vi "Validate Attributes JSON.vi"(6 "$Path":string="$.Attributes", 8 "error in":errorcluster, 10 "Cluster in":variant, 11 "<JSON>":string) -> (0 "error out":errorcluster, 2 "<JSON>":string)   [LabVIEW 2023]
uses:
  b690fbb4-b114-4137-a40c-faf688a51290.vi
  <vilib>/JDP Science/JSONtext/Next JSON Value.vi
  <vilib>/JDP Science/JSONtext/String Subset.vi
  <vilib>/JDP Science/JSONtext/Parsing/Advance past next JSON Value (inlined COPY).vi
  <vilib>/JDP Science/JSONtext/Parsing/Advance past whitespace.vi
  <vilib>/JDP Science/JSONtext/Parsing/Advance past String.vi
  <vilib>/JDP Science/JSONtext/Parsing/Advance past Number.vi
  <vilib>/JDP Science/JSONtext/Parsing/Advance past Line Ending.vi
  <vilib>/JDP Science/JSONtext/Variant to JSON Text.vi
  <vilib>/JDP Science/JSONtext/Parsing/Parse Full Path or Item Name.vi
  <vilib>/JDP Science/JSONtext/Parsing/Advance past Array.vi
  <vilib>/JDP Science/JSONtext/Parsing/Advance past Object.vi
  <vilib>/JDP Science/JSONtext/support/Error Cluster From Code.vi
  <vilib>/JDP Science/JSONtext/Offset/Find Item Locations by Path.vi
  <vilib>/JDP Science/JSONtext/LVClass Serializer/JSONtext LVClass Serializer.lvclass
  <vilib>/JDP Science/JSONtext/JSONtext.lvlib
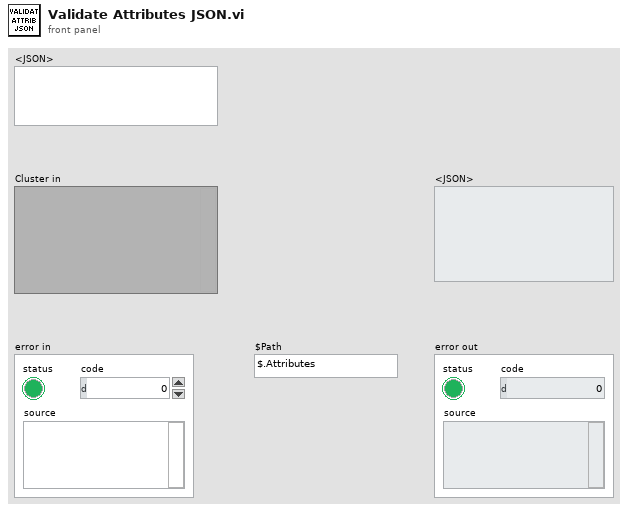
[diagram p1: front panel]
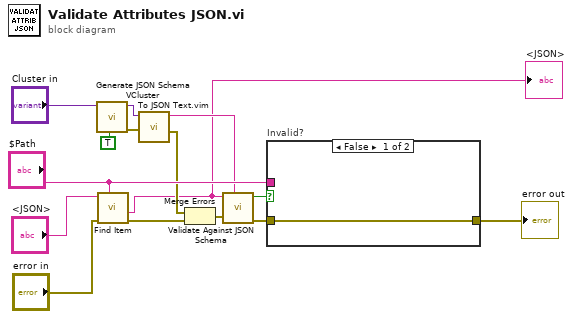
[diagram p0: block diagram]
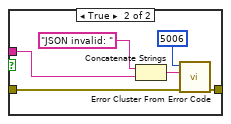
[diagram p2: hidden frame]
diagram:
  n1 = call "Generate JSON Schema VCluster.vi"("strict?"=TRUE, "type"="Cluster in") -> ("error out"=w6:errorcluster, "json schema cluster"=w5:variant)  [unwired: 8 in]
  n2 = call <vilib>:"Find Item.vi"("$Path or Item Name"="$Path", "error in (no error)"="error in", "JSON"="<JSON>") -> ("error out"=w11:errorcluster, "<JSON>"=w1:string)  [unwired: 5 in, 2 out]
  "<JSON>" <- w1
  n3 = call "To JSON Text.vim"("error in (no error)"=w6, "Anything"=w5) -> ("error out"=w8:errorcluster, "<JSON>"=w9:string)  [unwired: 8 in]
  n4 = Merge Errors(w8, w11) -> (w7:errorcluster)
  n5 = call <vilib>:"Validate Against JSON Schema.vi"("JSON Schema"=w9, "error in (no error)"=w7, "JSON"=w1) -> ("error out"=w12:errorcluster, "Invalid"=w14:bool)  [unwired: 4 in, 3 out]
  n6 = case "Invalid?" shown="False" w14 {
    tunnel: w12 -> [w16 w22]
    tunnel: [w16 w21] -> w13
    tunnel: "$Path" -> [_ w17]
    frame False {
    }
    frame True {
      n7 = Concatenate Strings("JSON invalid: " ("string"), w17) -> (w19:string)
      n8 = call <vilib>:"Error Cluster From Error Code.vi"("error in (no error)"=w22, "error message (\"\")"=w19, "error code (0)"=5006) -> ("error out"=w21:errorcluster)  [unwired: 6 in]
    }
  }
  "error out" <- w13
